vi "Stoerungen (193-256) - PNS.vi"(8 "Fehler (Eingang)":errorcluster caption="Fehler (Eingang, kein Fehler)") -> (0 "Fehler (Ausgang)":errorcluster, 3 "Störungen 193-256":u64)   [LabVIEW 2020, in "Stoerungen.lvlib"]
uses:
  Stoerungen.lvlib
  Seiten/System Einstellungen V2/Aktioen FGV System.ctl
  cRIO/Stoermeldungen/Stoerungen 193-256.ctl
  PNS/Parameternamen PNS.ctl
  Stoerungen Messgeraet/Aktionen Kommunikation Stoerung.ctl
  PNS/Aktionen FGV Istwerte.ctl
  PNS/Aktionen FGV Loopkennung.ctl
  Allgemein/Aktion FGV Aufheizphase.ctl
  cRIO/Stoermeldungen/Stoermeldungen.lvlib
  PNS/PNS.lvlib
  Seiten/System Einstellungen V2/System Einstellungen V2.lvlib
  Allgemein/allgemeine Sub-VIs.lvlib
panel:
  # "Störmeldungen PNS (193-256)"
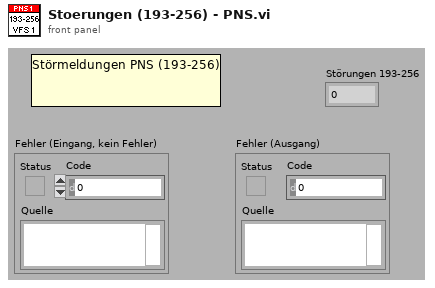
[diagram p1: front panel]
types:
  T1 = typedef "System Einstellungen V2.lvlib/Aktioen FGV System.ctl" = enum16{"lesen", "laden", "speichern", "Optionen schreiben", "Zeitstempel", "Reset BMP", "Reset SQP", "Wartung", "Werkseinstellung"}
  T2 = typedef "System Einstellungen V2.lvlib/Optionen.ctl" = cluster{"Störmeldep.":bool, "Betriebszustände":bool, "AK in ppm":bool, "log Cal-Gas":bool, "log 0-Gas":bool, "Durchflusssensor 0-5V":bool, "PNS?":bool, "Mit N2 spülen":bool, "TRE08":bool, "Amium 10-Fach":bool, "Verticale Scrollbar aktiv":bool, "Loggingtakt":bool, "AK Rezeptwechsel gleich wie MKS":bool, "NG ECO":bool}
  T3 = typedef "allgemeine Sub-VIs.lvlib/Aktion FGV Aufheizphase.ctl" = enum16{"init", "lesen", "PNS Filterblock", "PNS HL1", "PNS HL2", "PNS HL3", "PNS HL4", "FTIR Messzelle", "HL 1", "HL 2", "HL zu FTIR", "auswerten"}
  T4 = typedef "PNS.lvlib/Aktionen FGV Loopkennung.ctl" = enum16{"lesen", "schreiben"}
  T5 = typedef "PNS.lvlib/Parameternamen PNS.ctl" = enum16{"Heizkreis 1", "Heizkreis 2", "Heizkreis 3", "Heizkreis 4", "Heizkreis 5", "Heizkreis 6", "Heizkreis 7", "Heizkreis 8"}
  T6 = typedef "PNS.lvlib/Aktionen FGV Istwerte.ctl" = enum16{"lesen", "initialisieren", "schreiben", "Störungen"}
  T7 = typedef "Stoerungen.lvlib/Aktionen Kommunikation Stoerung.ctl" = enum16{"lesen", "init", "FT-IR Komm", "FT-IR Betriebsart", "FT-IR Hintergrund", "cRIO Komm", "PNS Komm", "Dichtheitstest", "Life Bit", "FTIR Komm AK", "PMA Komm", "FID Komm", "PMA Cal", "FID Ch4 Cal", "FID THC Cal", "Cal Timeout", "VFS 1 Komm", "VFS 2 Komm", "VFS 3 Komm", "VFS 4 Komm", "TRE 08 Komm", "CG-Test vorzeitig", "CG-Test Span 1", "CG-Test Span 2", "CG-Test Span 3", "CG-Test Messgas", "CG-Test löschen", "Test", "Amium AK", "AK Recept konfig", "AK Name konfig", "AK EKFG konfig"}
  T8 = typedef "Stoermeldungen.lvlib/Stoerungen 193-256.ctl" = cluster{"ERR. 193":bool, "ERR. 194":bool, "ERR. 195":bool, "ERR. 196":bool, "ERR. 197":bool, "ERR. 198":bool, "ERR. 199":bool, "ERR. 200":bool, "ERR. 201":bool, "ERR. 202":bool, "ERR. 203":bool, "ERR. 204":bool, "ERR. 205":bool, "ERR. 206":bool, "ERR. 207":bool, "ERR. 208":bool, "ERR. 209":bool, "ERR. 210":bool, "ERR. 211":bool, "ERR. 212":bool, "ERR. 213":bool, "ERR. 214":bool, "ERR. 215":bool, "ERR. 216":bool, "ERR. 217":bool, "ERR. 218":bool, "ERR. 219":bool, "ERR. 220":bool, "ERR. 221":bool, "ERR. 222":bool, "ERR. 223":bool, "ERR. 224":bool, "ERR. 225":bool, "ERR. 226":bool, "ERR. 227":bool, "ERR. 228":bool, "ERR. 229":bool, "ERR. 230":bool, "ERR. 231":bool, "ERR. 232":bool, "ERR. 233":bool, "ERR. 234":bool, "ERR. 235":bool, "ERR. 236":bool, "ERR. 237":bool, "ERR. 238":bool, "ERR. 239":bool, "ERR. 240":bool, "ERR. 241":bool, "ERR. 242":bool, "ERR. 243":bool, "ERR. 244":bool, "ERR. 245":bool, "ERR. 246":bool, "ERR. 247":bool, "ERR. 248":bool, "ERR. 249":bool, "ERR. 250":bool, "ERR. 251":bool, "ERR. 252":bool, "ERR. 253":bool, "ERR. 254":bool, "ERR. 255":bool, "ERR. 256":bool}
  T9 = typedef "PNS.lvlib/PNS Geraetekennung.ctl" = cluster{"Loops":string[], "Gerätetype":string, "Loopkennung":u16[], "Seriennummer":string, "Geraetekennung":u16, "SoftWare Version":string, "LP Kennung":u16}
  T10 = typedef "Steuerung PNS.lvclass/Regler.ctl" = cluster{"Istwert":i16, "Sollwert":i16, "Alarm MIN":i16, "Alarm MAX":i16, "Regler sperren":i16, "Analog Ausgang":i16}[]
  T11 = cluster{"Istwert":i16, "Sollwert":i16, "Alarm MIN":i16, "Alarm MAX":i16, "Regler sperren":i16, "Analog Ausgang":i16}
  T12 = typedef "Stoerungen.lvlib/Stoerungen Messgeraete.ctl" = cluster{"FT-IR Komm":bool, "FT-IR Betriebsart":bool, "FT-IR Hintergrundscan":bool, "Dichtheitstest":bool, "cRIO Komm":bool, "PNS Komm":bool, "Life Bit":bool, "FT-IR AK Komm":bool, "PMA Komm":bool, "FID Komm":bool, "PMA Cal":bool, "FID CH4 Cal":bool, "FID THC Cal":bool, "Cal Timeout":bool, "VFS 1 Komm":bool, "VFS 2 Komm":bool, "VFS 3 Komm":bool, "VFS 4 Komm":bool, "TRE 08 Komm":bool, "CG-Test":bool, "CG-Test 1":bool, "CG-Test 2":bool, "CG-Test 3":bool, "Messgas - Eingang":bool, "Amium AK Komm":bool, "AK Rezept nicht konfiguriert ":bool, "AK Name nicht konfiguriert":bool, "AK EKFG nicht konfiguriert":bool}
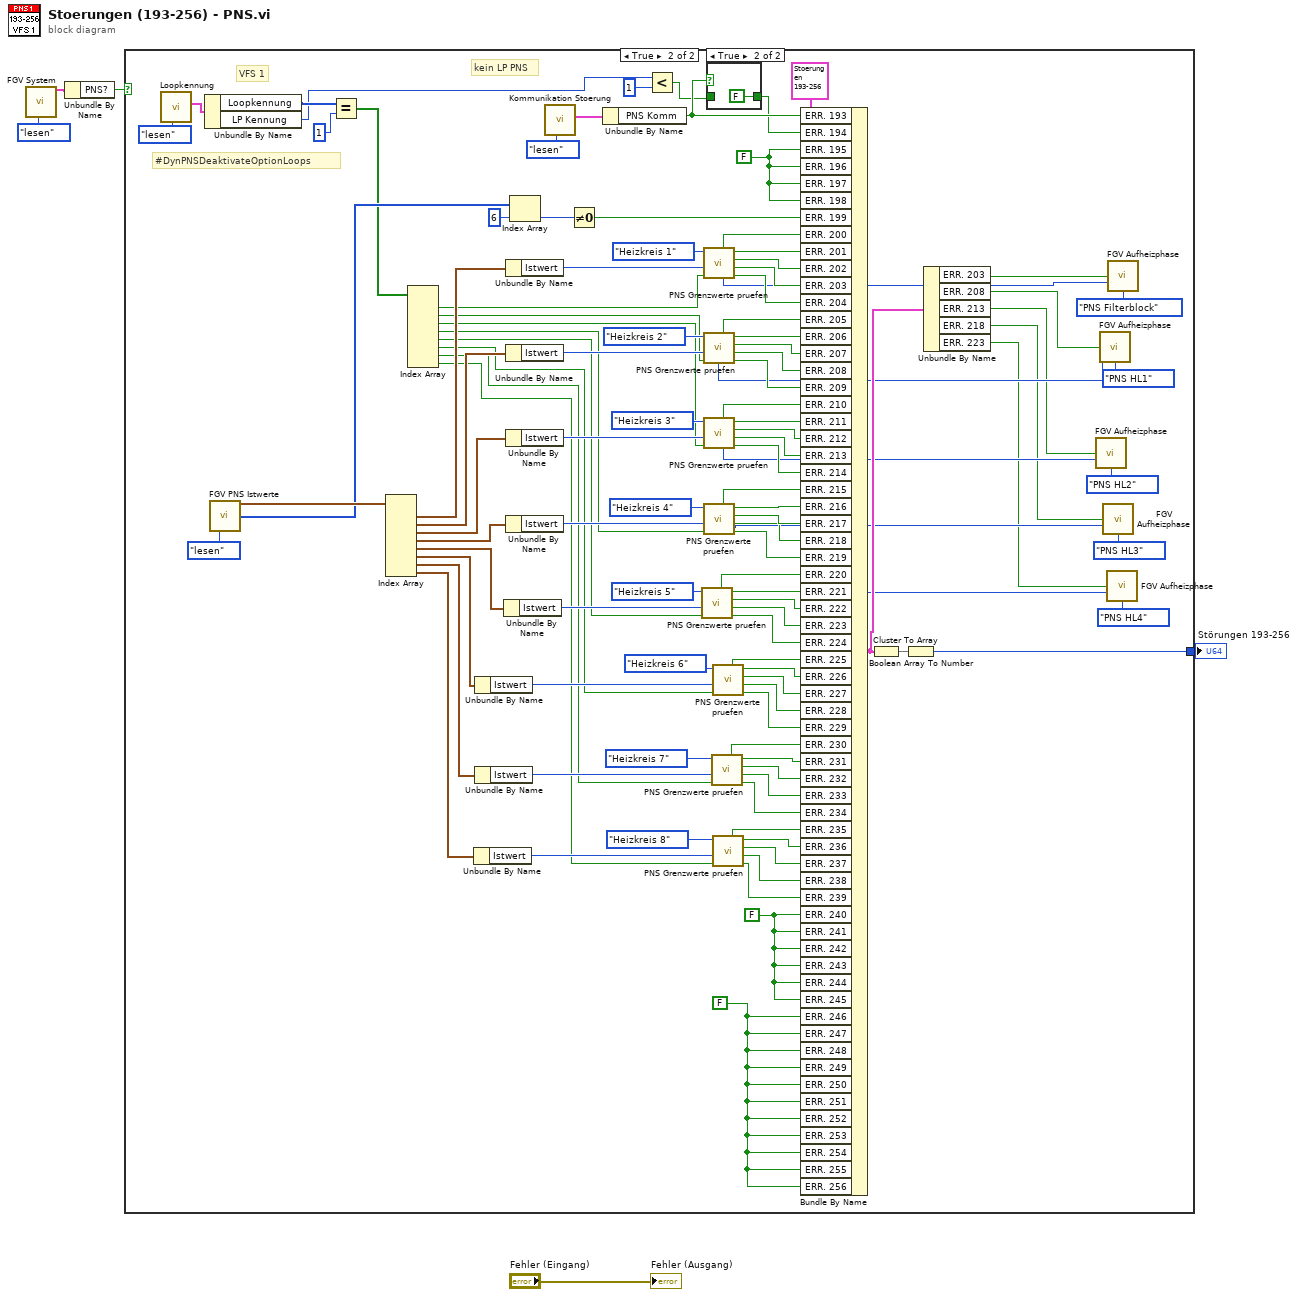
[diagram p0: block diagram]
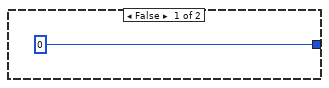
[diagram p2: hidden frame]
diagram:
  n1 = call "FGV System.vi"("Aktionen"=Aktioen_FGV_System."lesen") -> ("Optionen"=w3:T2)  [unwired: 12 in, 6 out]
  n2 = Unbundle By Name(w3) -> ("PNS?"=w1:bool)
  n3 = case shown="True" w1 {
    tunnel: [u64 0 w82] -> w4
    frame False {
    }
    frame True {
      w81 = FALSE ("ERR. 240")
      w86 = FALSE ("ERR. 194")
      w25 = FALSE ("ERR. 194")
      # "kein LP PNS"
      # "#DynPNSDeaktivateOptionLoops"
      # "VFS 1"
      n4 = call "Loopkennung.vi"("Aktion"=Aktionen_FGV_Loopkennung."lesen") -> ("LoopGeraetekennung"=w40:T9)  [unwired: 9 in, 1 out]
      n5 = Unbundle By Name(w40) -> ("Loopkennung"=w39:u16[], "LP Kennung"=w11:u16)
      n6 = call "FGV PNS Istwerte.vi"("Aktionen"=Aktionen_FGV_Istwerte."lesen") -> ("Regler"=w116:T10, "UsrVal"=w42:u16[])  [unwired: 11 in, 2 out]
      n7 = Equal?(x=w39, y=1 ("Index")) -> (x = y?=w37:bool[])
      n8 = Index Array(array=w116) -> (element #1=w115:T11, element #2=w113:T11, element #3=w112:T11, element #4=w111:T11, element #5=w75:T11, element #6=w69:T11, element #7=w68:T11, element #8=w67:T11)  [unwired: 8 in]
      n9 = Index Array(array=w37) -> (element #1=w36:bool, element #2=w35:bool, element #3=w34:bool, element #4=w33:bool, element #5=w32:bool, element #6=w31:bool, element #7=w30:bool, element #8=w29:bool)  [unwired: 8 in]
      n10 = Unbundle By Name(w67) -> ("Istwert"=w46:i16)
      n11 = Unbundle By Name(w69) -> ("Istwert"=w47:i16)
      n12 = Unbundle By Name(w68) -> ("Istwert"=w48:i16)
      n13 = Unbundle By Name(w75) -> ("Istwert"=w44:i16)
      n14 = Unbundle By Name(w115) -> ("Istwert"=w114:i16)
      n15 = Unbundle By Name(w113) -> ("Istwert"=w78:i16)
      n16 = Unbundle By Name(w112) -> ("Istwert"=w110:i16)
      n17 = Unbundle By Name(w111) -> ("Istwert"=w109:i16)
      n18 = Index Array(array=w42, index=6 ("Index")) -> (element=w84:u16)
      n19 = call "Kommunikation Stoerung.vi"("Aktionen"=Aktionen_Kommunikation_Stoerung."lesen") -> ("Störung Messgerät"=w88:T12)  [unwired: 10 in]
      n20 = Not Equal To 0?(x=w84) -> (x != 0?=w83:bool)
      n21 = Unbundle By Name(w88) -> ("PNS Komm"=w9:bool)
      n22 = Less?(x=w11, y=u16 1) -> (x < y?=w8:bool)
      n23 = call "PNS Grenzwerte pruefen.vi"("Option"=w32, "Wert"=w44, "Parameternamen PNS"=Parameternamen_PNS."Heizkreis 5") -> ("AbschMax"=w70:bool, "AbschMin"=w71:bool, "WarnMax"=w72:bool, "WarnMin"=w73:bool, "Regler"=w12:u16, "F.Br."=w74:bool)  [unwired: 3 in]
      n24 = call "PNS Grenzwerte pruefen.vi"("Option"=w36, "Wert"=w114, "Parameternamen PNS"=Parameternamen_PNS."Heizkreis 1") -> ("AbschMax"=w104:bool, "AbschMin"=w105:bool, "WarnMax"=w106:bool, "WarnMin"=w107:bool, "Regler"=w23:u16, "F.Br."=w108:bool)  [unwired: 3 in]
      n25 = call "PNS Grenzwerte pruefen.vi"("Option"=w35, "Wert"=w78, "Parameternamen PNS"=Parameternamen_PNS."Heizkreis 2") -> ("AbschMax"=w99:bool, "AbschMin"=w100:bool, "WarnMax"=w101:bool, "WarnMin"=w102:bool, "Regler"=w22:u16, "F.Br."=w103:bool)  [unwired: 3 in]
      n26 = call "PNS Grenzwerte pruefen.vi"("Option"=w34, "Wert"=w110, "Parameternamen PNS"=Parameternamen_PNS."Heizkreis 3") -> ("AbschMax"=w94:bool, "AbschMin"=w95:bool, "WarnMax"=w96:bool, "WarnMin"=w97:bool, "Regler"=w19:u16, "F.Br."=w98:bool)  [unwired: 3 in]
      n27 = call "PNS Grenzwerte pruefen.vi"("Option"=w33, "Wert"=w109, "Parameternamen PNS"=Parameternamen_PNS."Heizkreis 4") -> ("AbschMax"=w89:bool, "AbschMin"=w90:bool, "WarnMax"=w91:bool, "WarnMin"=w92:bool, "Regler"=w15:u16, "F.Br."=w93:bool)  [unwired: 3 in]
      n28 = case shown="True" w9 {
        tunnel: w8 -> [w119 _]
        tunnel: [w119 FALSE] -> w7
        frame False {
        }
        frame True {
        }
      }
      n29 = call "PNS Grenzwerte pruefen.vi"("Option"=w30, "Wert"=w48, "Parameternamen PNS"=Parameternamen_PNS."Heizkreis 7") -> ("AbschMax"=w57:bool, "AbschMin"=w58:bool, "WarnMax"=w59:bool, "WarnMin"=w60:bool, "F.Br."=w61:bool)  [unwired: 3 in, 1 out]
      n30 = call "PNS Grenzwerte pruefen.vi"("Option"=w31, "Wert"=w47, "Parameternamen PNS"=Parameternamen_PNS."Heizkreis 6") -> ("AbschMax"=w62:bool, "AbschMin"=w63:bool, "WarnMax"=w64:bool, "WarnMin"=w65:bool, "F.Br."=w66:bool)  [unwired: 3 in, 1 out]
      n31 = call "PNS Grenzwerte pruefen.vi"("Option"=w29, "Wert"=w46, "Parameternamen PNS"=Parameternamen_PNS."Heizkreis 8") -> ("AbschMax"=w52:bool, "AbschMin"=w53:bool, "WarnMax"=w54:bool, "WarnMin"=w55:bool, "F.Br."=w56:bool)  [unwired: 3 in, 1 out]
      n32 = Bundle By Name(cluster=T8 {"ERR. 193"=FALSE, "ERR. 194"=FALSE, "ERR. 195"=FALSE, "ERR. 196"=FALSE, "ERR. 197"=FALSE, "ERR. 198"=FALSE, "ERR. 199"=FALSE, "ERR. 200"=FALSE, "ERR. 201"=FALSE, "ERR. 202"=FALSE, "ERR. 203"=FALSE, "ERR. 204"=FALSE, "ERR. 205"=FALSE, "ERR. 206"=FALSE, "ERR. 207"=FALSE, "ERR. 208"=FALSE, "ERR. 209"=FALSE, "ERR. 210"=FALSE, "ERR. 211"=FALSE, "ERR. 212"=FALSE, "ERR. 213"=FALSE, "ERR. 214"=FALSE, "ERR. 215"=FALSE, "ERR. 216"=FALSE, "ERR. 217"=FALSE, "ERR. 218"=FALSE, "ERR. 219"=FALSE, "ERR. 220"=FALSE, "ERR. 221"=FALSE, "ERR. 222"=FALSE, "ERR. 223"=FALSE, "ERR. 224"=FALSE, "ERR. 225"=FALSE, "ERR. 226"=FALSE, "ERR. 227"=FALSE, "ERR. 228"=FALSE, "ERR. 229"=FALSE, "ERR. 230"=FALSE, "ERR. 231"=FALSE, "ERR. 232"=FALSE, "ERR. 233"=FALSE, "ERR. 234"=FALSE, "ERR. 235"=FALSE, "ERR. 236"=FALSE, "ERR. 237"=FALSE, "ERR. 238"=FALSE, "ERR. 239"=FALSE, "ERR. 240"=FALSE, "ERR. 241"=FALSE, "ERR. 242"=FALSE, "ERR. 243"=FALSE, "ERR. 244"=FALSE, "ERR. 245"=FALSE, "ERR. 246"=FALSE, "ERR. 247"=FALSE, "ERR. 248"=FALSE, "ERR. 249"=FALSE, "ERR. 250"=FALSE, "ERR. 251"=FALSE, "ERR. 252"=FALSE, "ERR. 253"=FALSE, "ERR. 254"=FALSE, "ERR. 255"=FALSE, "ERR. 256"=FALSE} ("STÖRUNGEN 193-256"), "ERR. 193"=w9, "ERR. 194"=w7, "ERR. 195"=w25, "ERR. 196"=w25, "ERR. 197"=w25, "ERR. 198"=w25, "ERR. 199"=w83, "ERR. 200"=w108, "ERR. 201"=w107, "ERR. 202"=w106, "ERR. 203"=w105, "ERR. 204"=w104, "ERR. 205"=w103, "ERR. 206"=w102, "ERR. 207"=w101, "ERR. 208"=w100, "ERR. 209"=w99, "ERR. 210"=w98, "ERR. 211"=w97, "ERR. 212"=w96, "ERR. 213"=w95, "ERR. 214"=w94, "ERR. 215"=w93, "ERR. 216"=w92, "ERR. 217"=w91, "ERR. 218"=w90, "ERR. 219"=w89, "ERR. 220"=w74, "ERR. 221"=w73, "ERR. 222"=w72, "ERR. 223"=w71, "ERR. 224"=w70, "ERR. 225"=w66, "ERR. 226"=w65, "ERR. 227"=w64, "ERR. 228"=w63, "ERR. 229"=w62, "ERR. 230"=w61, "ERR. 231"=w60, "ERR. 232"=w59, "ERR. 233"=w58, "ERR. 234"=w57, "ERR. 235"=w56, "ERR. 236"=w55, "ERR. 237"=w54, "ERR. 238"=w53, "ERR. 239"=w52, "ERR. 240"=w81, "ERR. 241"=w81, "ERR. 242"=w81, "ERR. 243"=w81, "ERR. 244"=w81, "ERR. 245"=w81, "ERR. 246"=w86, "ERR. 247"=w86, "ERR. 248"=w86, "ERR. 249"=w86, "ERR. 250"=w86, "ERR. 251"=w86, "ERR. 252"=w86, "ERR. 253"=w86, "ERR. 254"=w86, "ERR. 255"=w86, "ERR. 256"=w86) -> (w27:T8)
      n33 = Cluster To Array(cluster=w27) -> (array=w118:bool[])
      n34 = Boolean Array To Number ("Boolesches Array nach Zahl")(Boolean array=w118) -> (number=w82:u64)
      n35 = Unbundle By Name(w27) -> ("ERR. 203"=w26:bool, "ERR. 208"=w21:bool, "ERR. 213"=w18:bool, "ERR. 218"=w16:bool, "ERR. 223"=w13:bool)
      n36 = call "FGV Aufheizphase.vi"("Error"=w18, "Aktiv/Inaktiv"=w19, "Aktion"=Aktion_FGV_Aufheizphase."PNS HL2") -> ()  [unwired: 10 in, 3 out]
      n37 = call "FGV Aufheizphase.vi"("Error"=w21, "Aktiv/Inaktiv"=w22, "Aktion"=Aktion_FGV_Aufheizphase."PNS HL1") -> ()  [unwired: 10 in, 3 out]
      n38 = call "FGV Aufheizphase.vi"("Error"=w16, "Aktiv/Inaktiv"=w15, "Aktion"=Aktion_FGV_Aufheizphase."PNS HL3") -> ()  [unwired: 10 in, 3 out]
      n39 = call "FGV Aufheizphase.vi"("Error"=w13, "Aktiv/Inaktiv"=w12, "Aktion"=Aktion_FGV_Aufheizphase."PNS HL4") -> ()  [unwired: 10 in, 3 out]
      n40 = call "FGV Aufheizphase.vi"("Error"=w26, "Aktiv/Inaktiv"=w23, "Aktion"=Aktion_FGV_Aufheizphase."PNS Filterblock") -> ()  [unwired: 10 in, 3 out]
    }
  }
  "Störungen 193-256" <- w4
  "Fehler (Ausgang)" <- "Fehler (Eingang)"
